vi "Process Sound.vi"(9 "Device":u32=2, 10 "Sampling \nFrequency (Hz)":dbl=44100.0, 11 "Time to Record (s)":dbl=1.0) -> (1 "Peak Frequency":dbl, 2 "Power Spectrum":waveform(dbl), 3 "Sound Data":cluster{dbl[], "Array":dbl[]})   [LabVIEW 2023]
uses:
  <vilib>/Analysis/NI_AALPro.lvlib
panel:
  out "Waveform Graph":waveform(dbl)(graph)
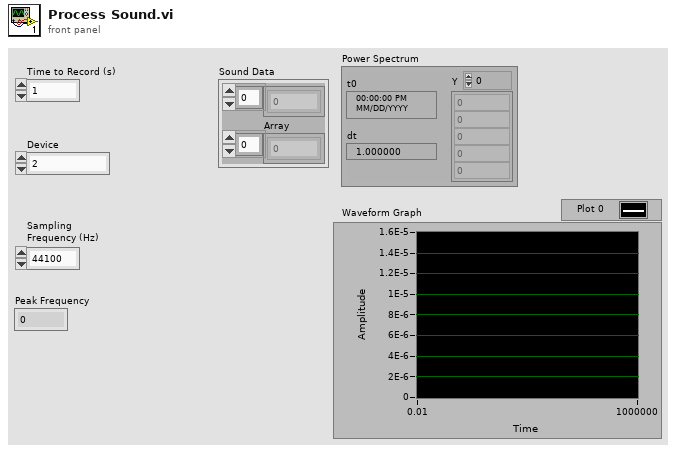
[diagram p1: front panel]
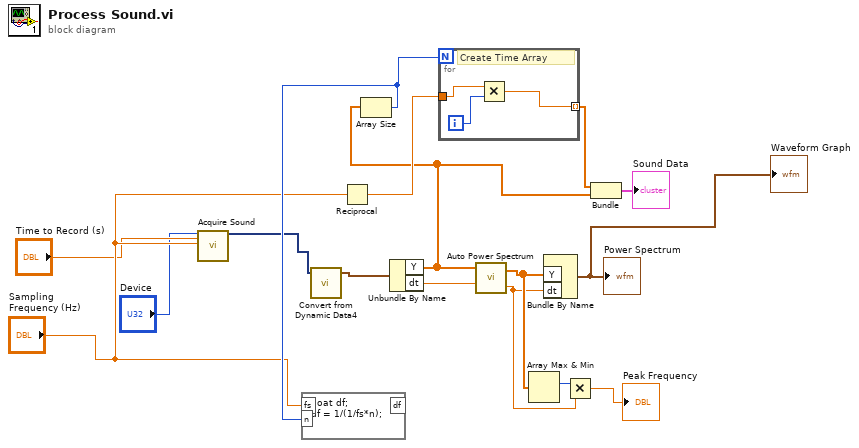
[diagram p0: block diagram]
diagram:
  n1 = call "Acquire Sound"("Device"="Device", "Duration (s)"="Time to Record (s)", "Sample rate (Hz)"="Sampling \nFrequency (Hz)") -> ("Data"=w7:dynamicdata)  [unwired: 15 in, 1 out]
  n2 = call "Convert from Dynamic Data4"("Dynamic Data Type"=w7) -> ("Waveform"=w6:waveform(dbl))  [unwired: 3 in]
  n3 = Reciprocal(x="Sampling \nFrequency (Hz)") -> (1/x=w10:dbl)
  n4 = Unbundle By Name(w6) -> ("Y"=w3:dbl[], "dt"=w5:dbl)
  n5 = Array Size(array=w3) -> (size(s)=w14:i32)
  n6 = formula code="float df;\ndf = 1/(1/fs*n);"("fs"="Sampling \nFrequency (Hz)", "n"=w14) -> ()  [unwired: 1 out]
  n7 = for {
    N: w14 -> [_]
    tunnel: w10 -> [w18]
    tunnel: [w17] -> w11 mode=indexing
    i -> [w19]
    # "Create Time Array"
    n8 = Multiply(x=w18, y=w19) -> (x*y=w17:dbl)
  }
  n9 = call <vilib>:"Auto Power Spectrum.vi"("dt"=w5, "Signal (V)"=w3) -> ("df"=w2:dbl, "Power Spectrum (V^2 rms)"=w4:dbl[])
  n10 = Array Max & Min(array=w4) -> (max index (indices)=w15:i32)  [unwired: 3 out]
  n11 = Bundle By Name("Y"=w4, "dt"=w2) -> (→"Power Spectrum" →"Waveform Graph":waveform(dbl))  [unwired: 1 in]
  n12 = Multiply(x=w15, y=w2) -> (x*y=→"Peak Frequency":dbl)
  n13 = Bundle(w11, "Y"=w3) -> (→"Sound Data":cluster{dbl[], "Y":dbl[]})  [unwired: 1 in]
